vi "Initalization_BK9201.vi"(3 "error in (no error)":errorcluster, 5 "Instrument In":refnum<visa-resource-name>) -> (0 "error out":errorcluster, 2 "Instrument Out":refnum<visa-resource-name>)   [LabVIEW 2022 SP3]
uses:
  <instrlib>/BK Precision 9200 Series/BK Precision 9200 Series.lvlib
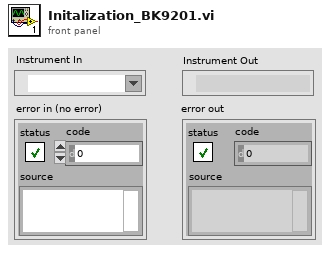
[diagram p1: front panel]
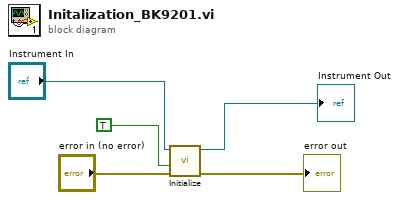
[diagram p0: block diagram]
diagram:
  n1 = call <instrlib>:"Initialize.vi"("error in (no error)"="error in (no error)", "Reset (True)"=TRUE, "VISA resource name"="Instrument In") -> ("error out"=→"error out":errorcluster, "VISA resource name out"=→"Instrument Out":refnum<visa-resource-name>)  [unwired: 7 in]
